vi "RunMeas.vi"(8 "error in (no error)":errorcluster, 11 "ChromaAcLoad in":refnum<class "ChromaAcLoad.lvclass">) -> (0 "error out":errorcluster, 2 "variant":variant, 3 "ChromaAcLoad out":refnum<class "ChromaAcLoad.lvclass">)   [LabVIEW 2018, in "AcPwrPlugins.lvlib" / "ChromaAcLoad.lvclass"]
doc: "This VI (may) initiate the measurement and retrieves the measurement value from the device."
uses:
  ChromaAcLoad.lvclass
  C:/Users/ico/Documents/Projects/NistPluggableModules/AcPwr/AcPwrPlugins/AcPwrBaseClass/AcPwrBase.lvclass
  AcPwrBaseClass/AcPwrBase.lvclass/AcPwrBase.ctl
  AcPwrBaseClass/Accessors/Read RefreshTime.vi
  <instrlib>/C63800/C63800.llb/C63800 M/F Overshoot Voltage.vi
  <instrlib>/C63800/C63800.llb/C63800 M/F Negative Peak Current.vi
  <instrlib>/C63800/C63800.llb/C63800 M/F Undershoot Voltage.vi
  <instrlib>/C63800/C63800.llb/C63800 M/F Apparent Power.vi
  <instrlib>/C63800/C63800.llb/C63800 M/F Power Reactive.vi
  <instrlib>/C63800/C63800.llb/C63800 M/F Power Factor.vi
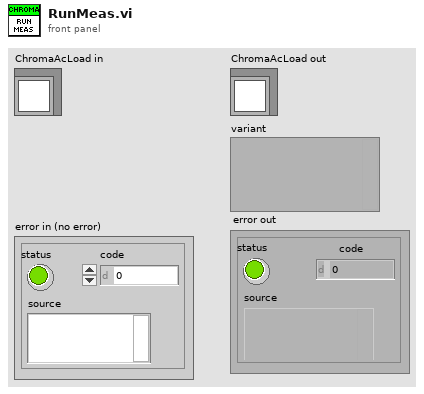
[diagram p1: front panel]
types:
  T1 = typedef "AcPwrPlugins.lvlib/ChromaAcLoad.lvclass/Measurements.ctl" = cluster{"Handle":string, "Name":string, "Enabled":bool, "Measurement Value":dbl, "Measurement Type":enum16{"Voltage (Vrms or V)", "Current (Arms or A)", "Power (W)", "Peak Voltage (V)", "Peak Current (A)", "Peak Power (W)", "Frequency (Hz)", "Resistance (Ohms)", "Voltage Overshoot (V)", "Positive Peak Current (A)", "Voltage Undershoot (V)", "Negative Peak Current (A)", "Apparent Power (VA)", "Reacitive Power (VAR)", "Voltage THD", "Power Factor", "Current's Crest Factor"}, "Hold Peak Current Measurement":bool, "btnMeasFetch":bool, "ProtectionStatusString":string}[]
  T2 = enum16{"Voltage (Vrms or V)", "Current (Arms or A)", "Power (W)", "Peak Voltage (V)", "Peak Current (A)", "Peak Power (W)", "Frequency (Hz)", "Resistance (Ohms)", "Voltage Overshoot (V)", "Positive Peak Current (A)", "Voltage Undershoot (V)", "Negative Peak Current (A)", "Apparent Power (VA)", "Reacitive Power (VAR)", "Voltage THD", "Power Factor", "Current's Crest Factor"}
  T3 = cluster{"Handle":string, "Name":string, "Enabled":bool, "Measurement Value":dbl, "Measurement Type":enum16{"Voltage (Vrms or V)", "Current (Arms or A)", "Power (W)", "Peak Voltage (V)", "Peak Current (A)", "Peak Power (W)", "Frequency (Hz)", "Resistance (Ohms)", "Voltage Overshoot (V)", "Positive Peak Current (A)", "Voltage Undershoot (V)", "Negative Peak Current (A)", "Apparent Power (VA)", "Reacitive Power (VAR)", "Voltage THD", "Power Factor", "Current's Crest Factor"}, "Hold Peak Current Measurement":bool, "btnMeasFetch":bool, "ProtectionStatusString":string}
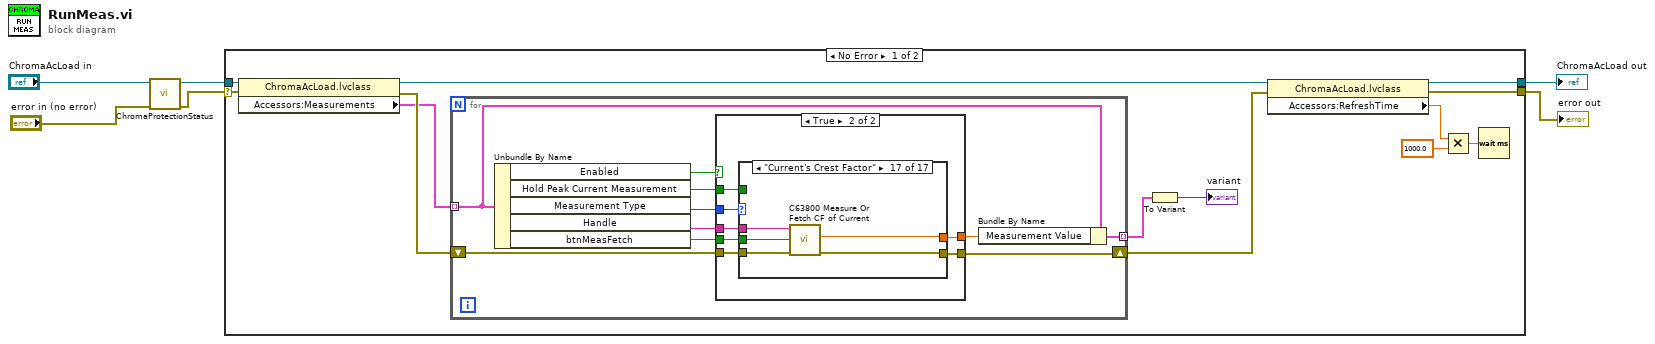
[diagram p0: block diagram]
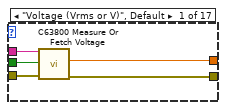
[diagram p3: hidden frame]
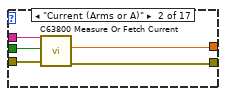
[diagram p4: hidden frame]
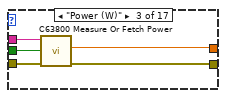
[diagram p5: hidden frame]
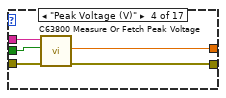
[diagram p6: hidden frame]
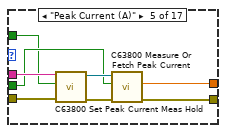
[diagram p7: hidden frame]
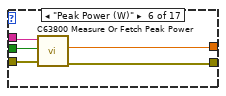
[diagram p8: hidden frame]
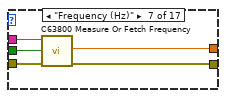
[diagram p9: hidden frame]
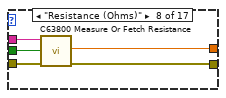
[diagram p10: hidden frame]
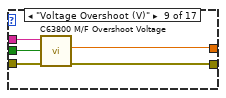
[diagram p11: hidden frame]
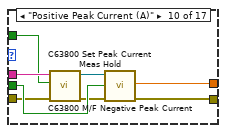
[diagram p12: hidden frame]
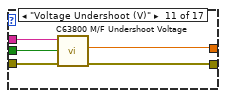
[diagram p13: hidden frame]
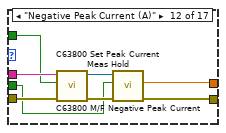
[diagram p14: hidden frame]
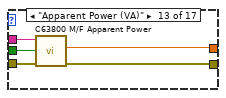
[diagram p15: hidden frame]
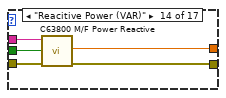
[diagram p16: hidden frame]
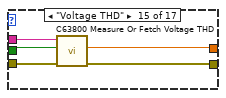
[diagram p17: hidden frame]
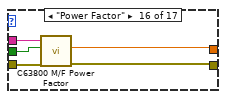
[diagram p18: hidden frame]
diagram:
  n1 = call "ChromaProtectionStatus.vi"("error in (no error)"="error in (no error)", "ChromaAcLoad in"="ChromaAcLoad in") -> ("error out"=w1:errorcluster, "ChromaAcLoad out"=w3:refnum<class "ChromaAcLoad.lvclass">)  [unwired: 8 in]
  n2 = case shown="No Error" w1 {
    selector: w1 -> [w11 w132]
    tunnel: [w17 w133] -> w6
    tunnel: [w16 w132] -> w5
    tunnel: w3 -> [w12 w133]
    frame No Error {
      n3 = property class="ChromaAcLoad.lvclass"(reference=w12, error in=w11) -> (reference out=w8:refnum<class "ChromaAcLoad.lvclass">, error out=w19:errorcluster, "Accessors:Measurements"=w18:T1)
      n4 = for {
        tunnel: w18 -> [w29] mode=indexing
        shift-right: [w25] -> w7
        shift-left: w19 -> [w27]
        tunnel: [w28] -> w10 mode=indexing
        n5 = Unbundle By Name(w29) -> ("Enabled"=w20:bool, "Hold Peak Current Measurement"=w22:bool, "Measurement Type"=w26:T2, "Handle"=w23:string, "btnMeasFetch"=w21:bool)
        n6 = case shown="True" w20 {
          tunnel: w27 -> [w30 w37]
          tunnel: w26 -> [_ w34]
          tunnel: [w30 w32] -> w25
          tunnel: [_ w31] -> w24
          tunnel: w23 -> [_ w36]
          tunnel: w22 -> [_ w33]
          tunnel: w21 -> [_ w35]
          frame False {
          }
          frame True {
            n7 = case shown="\"Current's Crest Factor\"" w34 {
              tunnel: w37 -> [w42 w45 w50 w57 w61 w68 w75 w80 w85 w88 w98 w102 w111 w116 w121 w126 w130]
              tunnel: w36 -> [w41 w44 w48 w55 w60 w66 w72 w76 w81 w87 w97 w101 w110 w112 w119 w125 w129]
              tunnel: w35 -> [w40 w43 w49 w56 w59 w67 w71 w77 w82 w91 w96 w100 w109 w113 w118 w124 w128]
              tunnel: w33 -> [_ _ _ _ w58 _ _ _ _ w86 _ w99 _ _ _ _ _]
              tunnel: [w39 w47 w52 w54 w65 w70 w74 w79 w84 w93 w95 w106 w108 w115 w120 w123 w131] -> w32
              tunnel: [w38 w46 w51 w53 w64 w69 w73 w78 w83 w92 w94 w105 w107 w114 w117 w122 w127] -> w31
              frame "Voltage (Vrms or V)", Default {
                n8 = call <instrlib>:"C63800 Measure Or Fetch Voltage.vi"("error in (no error)"=w42, "Query Type"=w40, "Instrument Handle"=w41) -> ("error out"=w39:errorcluster, "Query Voltage"=w38:dbl)  [unwired: 6 in, 1 out]
              }
              frame "Current (Arms or A)" {
                n9 = call <instrlib>:"C63800 Measure Or Fetch Current.vi"("error in (no error)"=w45, "Query Type"=w43, "Instrument Handle"=w44) -> ("error out"=w47:errorcluster, "Query Current"=w46:dbl)  [unwired: 6 in, 1 out]
              }
              frame "Power (W)" {
                n10 = call <instrlib>:"C63800 Measure Or Fetch Power.vi"("error in (no error)"=w50, "Query Type"=w49, "Instrument Handle"=w48) -> ("error out"=w52:errorcluster, "Query Power"=w51:dbl)  [unwired: 6 in, 1 out]
              }
              frame "Peak Voltage (V)" {
                n11 = call <instrlib>:"C63800 Measure Or Fetch Peak Voltage.vi"("error in (no error)"=w57, "Query Type"=w56, "Instrument Handle"=w55) -> ("error out"=w54:errorcluster, "Query Peak Voltage"=w53:dbl)  [unwired: 6 in, 1 out]
              }
              frame "Peak Current (A)" {
                n12 = call <instrlib>:"C63800 Set Peak Current Meas Hold.vi"("error in (no error)"=w61, "Hold State"=w58, "Instrument Handle"=w60) -> ("error out"=w63:errorcluster, "Instrument Handle out"=w62:refnum<k15>)  [unwired: 7 in]
                n13 = call <instrlib>:"C63800 Measure Or Fetch Peak Current.vi"("error in (no error)"=w63, "Query Type"=w59, "Instrument Handle"=w62) -> ("error out"=w65:errorcluster, "Query Peak Current"=w64:dbl)  [unwired: 6 in, 1 out]
              }
              frame "Peak Power (W)" {
                n14 = call <instrlib>:"C63800 Measure Or Fetch Peak Power.vi"("error in (no error)"=w68, "Query Type"=w67, "Instrument Handle"=w66) -> ("error out"=w70:errorcluster, "Query Peak Power"=w69:dbl)  [unwired: 6 in, 1 out]
              }
              frame "Frequency (Hz)" {
                n15 = call <instrlib>:"C63800 Measure Or Fetch Frequency.vi"("error in (no error)"=w75, "Query Type"=w71, "Instrument Handle"=w72) -> ("error out"=w74:errorcluster, "Query Frequency"=w73:dbl)  [unwired: 6 in, 1 out]
              }
              frame "Resistance (Ohms)" {
                n16 = call <instrlib>:"C63800 Measure Or Fetch Resistance.vi"("error in (no error)"=w80, "Query Type"=w77, "Instrument Handle"=w76) -> ("error out"=w79:errorcluster, "Query Resistance"=w78:dbl)  [unwired: 6 in, 1 out]
              }
              frame "Voltage Overshoot (V)" {
                n17 = call "C63800 M/F Overshoot Voltage.vi"("error in (no error)"=w85, "Query Type"=w82, "Instrument Handle"=w81) -> ("error out"=w84:errorcluster, "Query Overshoot Voltage"=w83:dbl)  [unwired: 6 in, 1 out]
              }
              frame "Positive Peak Current (A)" {
                n18 = call <instrlib>:"C63800 Set Peak Current Meas Hold.vi"("error in (no error)"=w88, "Hold State"=w86, "Instrument Handle"=w87) -> ("error out"=w90:errorcluster, "Instrument Handle out"=w89:refnum<k15>)  [unwired: 7 in]
                n19 = call "C63800 M/F Negative Peak Current.vi"("error in (no error)"=w90, "Query Type"=w91, "Instrument Handle"=w89) -> ("error out"=w93:errorcluster, "Query Negative Peak Current"=w92:dbl)  [unwired: 6 in, 1 out]
              }
              frame "Voltage Undershoot (V)" {
                n20 = call "C63800 M/F Undershoot Voltage.vi"("error in (no error)"=w98, "Query Type"=w96, "Instrument Handle"=w97) -> ("error out"=w95:errorcluster, "Query Undershoot Voltage"=w94:dbl)  [unwired: 6 in, 1 out]
              }
              frame "Negative Peak Current (A)" {
                n21 = call <instrlib>:"C63800 Set Peak Current Meas Hold.vi"("error in (no error)"=w102, "Hold State"=w99, "Instrument Handle"=w101) -> ("error out"=w104:errorcluster, "Instrument Handle out"=w103:refnum<k15>)  [unwired: 7 in]
                n22 = call "C63800 M/F Negative Peak Current.vi"("error in (no error)"=w104, "Query Type"=w100, "Instrument Handle"=w103) -> ("error out"=w106:errorcluster, "Query Negative Peak Current"=w105:dbl)  [unwired: 6 in, 1 out]
              }
              frame "Apparent Power (VA)" {
                n23 = call "C63800 M/F Apparent Power.vi"("error in (no error)"=w111, "Query Type"=w109, "Instrument Handle"=w110) -> ("error out"=w108:errorcluster, "Query Apparent Power"=w107:dbl)  [unwired: 6 in, 1 out]
              }
              frame "Reacitive Power (VAR)" {
                n24 = call "C63800 M/F Power Reactive.vi"("error in (no error)"=w116, "Query Type"=w113, "Instrument Handle"=w112) -> ("error out"=w115:errorcluster, "Query Power Reactive"=w114:dbl)  [unwired: 6 in, 1 out]
              }
              frame "Voltage THD" {
                n25 = call <instrlib>:"C63800 Measure Or Fetch Voltage THD.vi"("error in (no error)"=w121, "Query Type"=w118, "Instrument Handle"=w119) -> ("error out"=w120:errorcluster, "Query Voltage THD"=w117:dbl)  [unwired: 6 in, 1 out]
              }
              frame "Power Factor" {
                n26 = call "C63800 M/F Power Factor.vi"("error in (no error)"=w126, "Query Type"=w124, "Instrument Handle"=w125) -> ("error out"=w123:errorcluster, "Query PF"=w122:dbl)  [unwired: 6 in, 1 out]
              }
              frame "Current's Crest Factor" {
                n27 = call <instrlib>:"C63800 Measure Or Fetch CF of Current.vi"("error in (no error)"=w130, "Query Type"=w128, "Instrument Handle"=w129) -> ("error out"=w131:errorcluster, "Query CF of Current"=w127:dbl)  [unwired: 6 in, 1 out]
              }
            }
          }
        }
        n28 = Bundle By Name(cluster=w29, "Measurement Value"=w24) -> (w28:T3)
      }
      n29 = To Variant(anything=w10) -> (Variant=→"variant":variant)
      n30 = property class="ChromaAcLoad.lvclass"(reference=w8, error in=w7) -> (reference out=w17:refnum<class "ChromaAcLoad.lvclass">, error out=w16:errorcluster, "Accessors:RefreshTime"=w13:dbl)
      n31 = Multiply(x=w13, y=1000.0) -> (x*y=w14:dbl)
      n32 = Wait (ms)(milliseconds to wait=w14) -> ()  [unwired: 1 out]
    }
    frame Error {
    }
  }
  "ChromaAcLoad out" <- w6
  "error out" <- w5
